vi "Launch Top Loop.vi"(8 "error in (no error)":errorcluster, 11 "PanelArray in":refnum<class "PanelArray.lvclass">) -> (0 "error out":errorcluster, 3 "PanelArray out":refnum<class "PanelArray.lvclass">)   [LabVIEW 2018, in "OOPanel.lvlib" / "PanelArray.lvclass"]
uses:
  PanelArray.lvclass
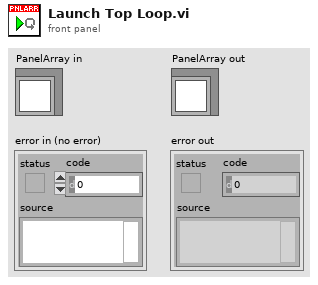
[diagram p1: front panel]
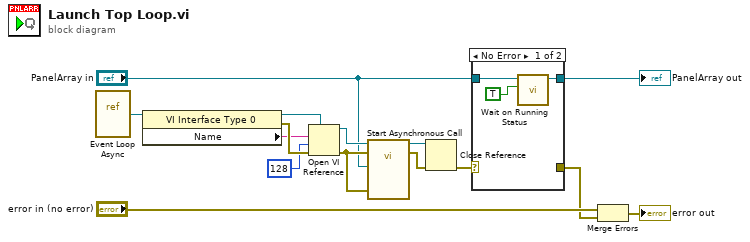
[diagram p0: block diagram]
diagram:
  n1 = vi-ref "Event Loop Async.vi"() -> (w14:refnum<vi>)
  n2 = property class="VI Interface Type 0"(reference=w14) -> (reference out=w12:refnum<vi>, error out=w15:errorcluster, "Name"=w13:string)  [unwired: 1 in]
  n3 = Open VI Reference(type specifier VI Refnum (for type only)=w12, vi path=w13, options=128, error in (no error)=w15) -> (vi reference=w11:refnum<vi>, error out=w10:errorcluster)  [unwired: 2 in]
  n4 = call-by-ref "Start Asynchronous Call"(reference=w11, error in=w10, 8:"error in (no error)"=w10, "PanelArray in"="PanelArray in") -> (reference out=w7:refnum<vi>, error out=w6:errorcluster)  [unwired: 10 in]
  n5 = Close Reference(reference=w7, error in (no error)=w6) -> (error out=w5:errorcluster)
  n6 = case shown="No Error" w5 {
    selector: w5 -> [_ w20]
    tunnel: "PanelArray in" -> [w18 w19]
    tunnel: [w16 w19] -> w3
    tunnel: [_ w20] -> w2
    frame No Error {
      n7 = call "Wait on Running Status.vi"("Running Value"=TRUE, "PanelArray in"=w18) -> ("PanelArray out"=w16:refnum<class "PanelArray.lvclass">)  [unwired: 8 in, 1 out]
    }
    frame Error {
    }
  }
  "PanelArray out" <- w3
  n8 = Merge Errors("error in (no error)", w2) -> (→"error out":errorcluster)
